vi "UI_Start Asychronous Call.vi"(8 "error in (no error)":errorcluster, 9 "DQMH Modules":T1, 10 "VI Refnum":refnum<vi>, 11 "User Event in":refnum<user-event>) -> (0 "error out":errorcluster, 3 "VI ref":refnum<vi>)   [LabVIEW 2025]
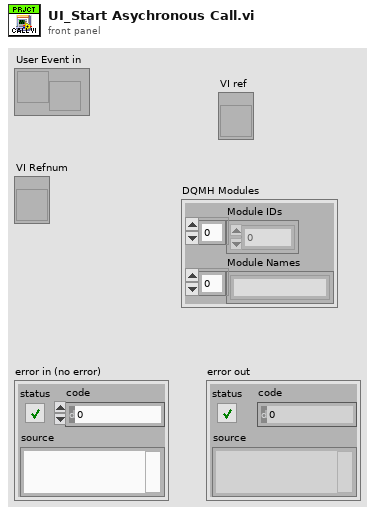
[diagram p1: front panel]
types:
  T1 = cluster{"Module IDs":i32[], "Module Names":string[]}
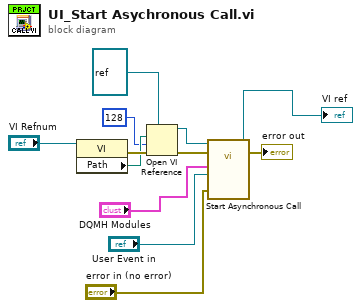
[diagram p0: block diagram]
diagram:
  n1 = property class="VI"(reference="VI Refnum") -> (error out=w9:errorcluster, "Path"=w5:path)  [unwired: 1 in, 1 out]
  n2 = Open VI Reference(type specifier VI Refnum (for type only)=refnum<vi> refnum, vi path=w5, options=128, error in (no error)=w9) -> (vi reference=w7:refnum<vi>, error out=w8:errorcluster)  [unwired: 2 in]
  n3 = call-by-ref "Start Asynchronous Call"(reference=w7, error in=w8, 8:"error in (no error)"="error in (no error)", "shutdown"="User Event in", "Modules"="DQMH Modules") -> (reference out=→"VI ref":refnum<vi>, error out=→"error out":errorcluster)  [unwired: 8 in, 1 out]
